vi "Add_APN.vi"(8 "error in (no error)":errorcluster, 11 "Add_APN":T1) -> (0 "error out":errorcluster, 3 "Output String":string)   [LabVIEW 2021]
uses:
  Controls/TCP_FGV.ctl
panel:
  # "SET,<add_apn>,<subscriber_N>,<no_of_apn>,<apn_name_i>,<qci_i>,<priority_level_i>,<no_of_dedicated_bearer_i_j>,<pcc_index_i_j>,<pcc_priority_index_i_j>,<mbr_dl_i_j>,<mbr_ul_i_j>,<gbr_dl_i_j>,<gbr_ul_i_j>"
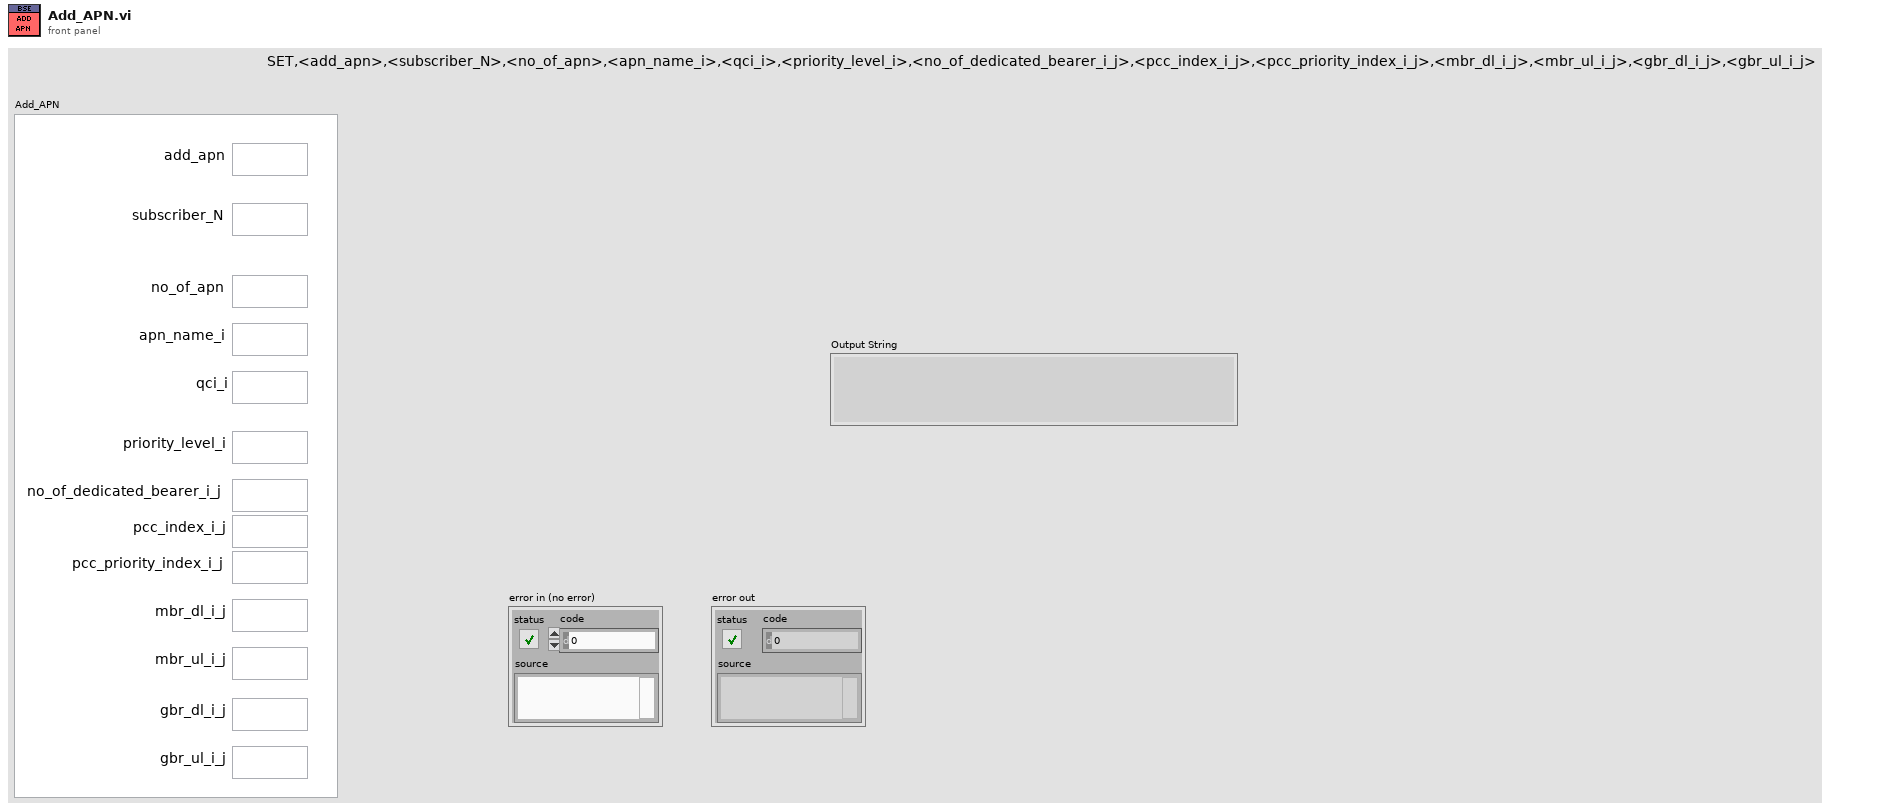
[diagram p1: front panel]
types:
  T1 = cluster{"add_apn":string, "subscriber_N":string, "no_of_apn":string, "apn_name_i":string, "qci_i":string, "priority_level_i":string, "no_of_dedicated_bearer_i_j":string, "pcc_index_i_j":string, "pcc_priority_index_i_j":string, "mbr_dl_i_j":string, "mbr_ul_i_j":string, "gbr_dl_i_j":string, "gbr_ul_i_j":string}
  T2 = typedef "TCP_FGV.ctl" = enum16{"Open", "Read", "Write", "Close"}
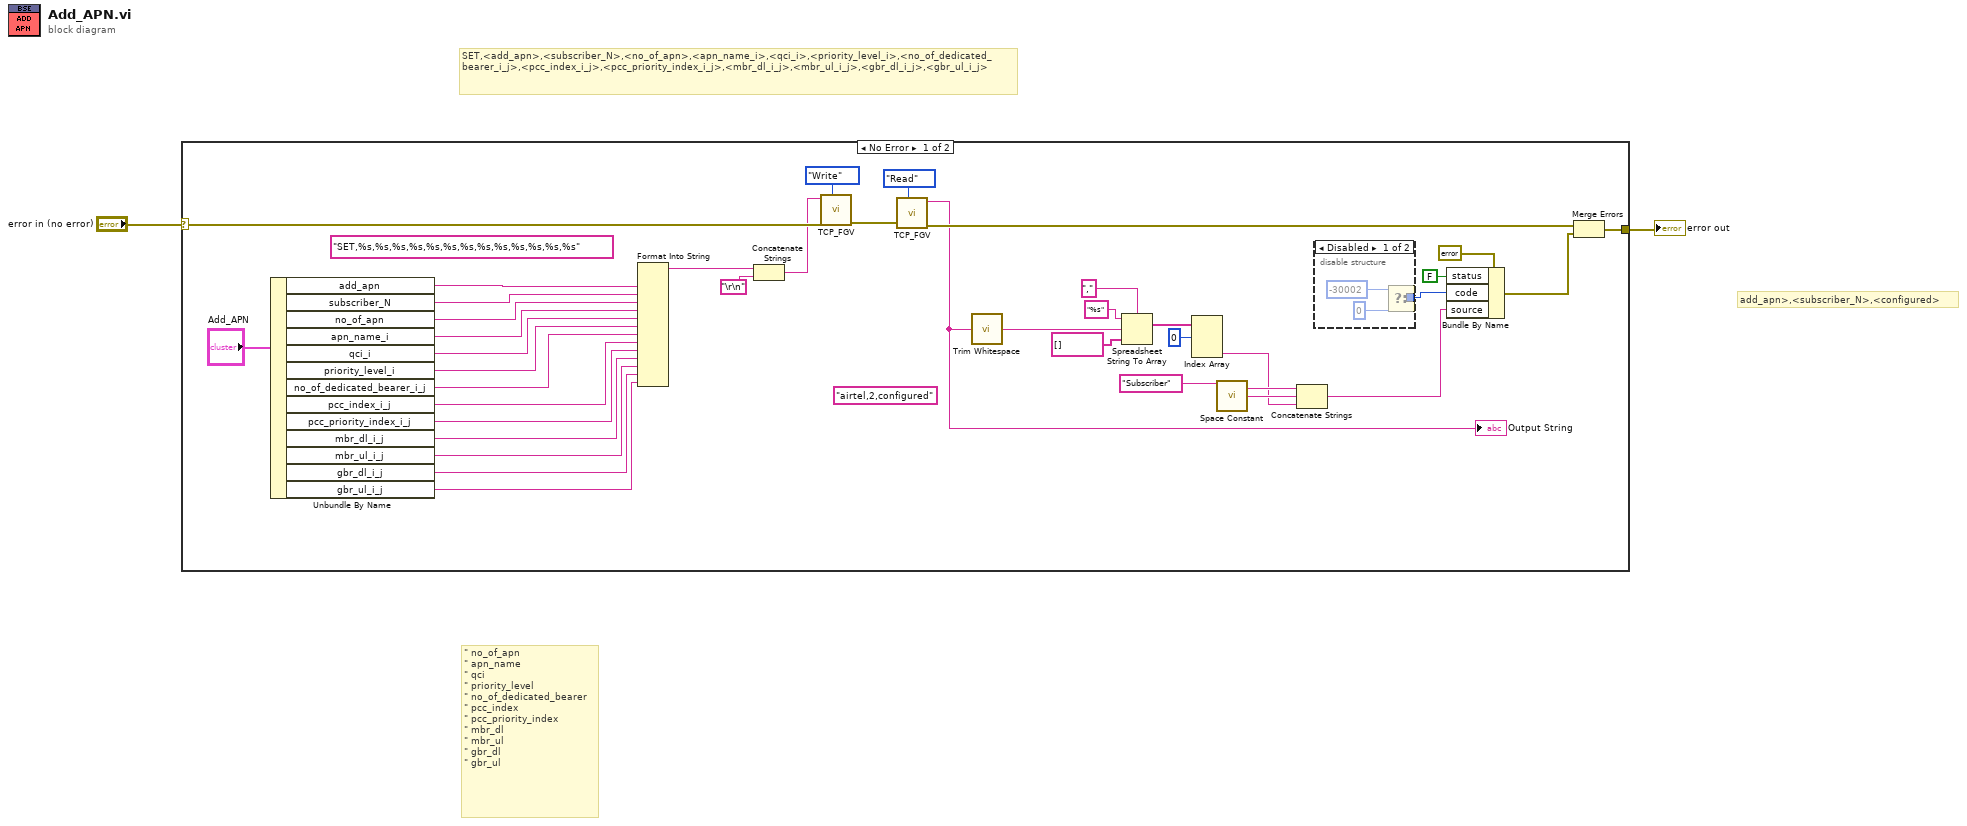
[diagram p0: block diagram]
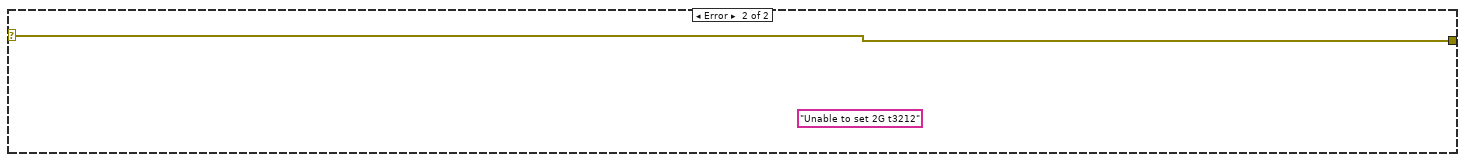
[diagram p3: hidden frame]
diagram:
  # "SET,<add_apn>,<subscriber_N>,<no_of_apn>,<apn_name_i>,<qci_i>,<priority_level_i>,<no_of_dedicated_bearer_i_j>,<pcc_index_i_j>,<pcc_priority_index_i_j>,<mbr_dl_i_j>,<mbr_ul_i_j>,<gbr_dl_i_j>,<gbr_ul_i_j>"
  # "\"\tno_of_apn \n\"\tapn_name\n\"\tqci\n\"\tpriority_level\n\"\tno_of_dedicated_bearer\n\"\tpcc_index\n\"\tpcc_priority_index\n\"\tmbr_dl\n\"\tmbr_ul\n\"\tgbr_dl\n\"\tgbr_ul"
  # "add_apn>,<subscriber_N>,<configured>"
  n1 = case shown="No Error" "error in (no error)" {
    selector: "error in (no error)" -> [w40 w44]
    tunnel: [w29 w44] -> w1
    frame No Error {
      (unwired) "airtel,2,configured" ("format string")
      (unwired) "SET,%s,%s,%s,%s,%s,%s,%s,%s,%s,%s,%s,%s,%s" ("format string")
      n2 = Unbundle By Name("Add_APN") -> ("add_apn"=w21:string, "subscriber_N"=w20:string, "no_of_apn"=w11:string, "apn_name_i"=w12:string, "qci_i"=w19:string, "priority_level_i"=w18:string, "no_of_dedicated_bearer_i_j"=w17:string, "pcc_index_i_j"=w9:string, "pcc_priority_index_i_j"=w8:string, "mbr_dl_i_j"=w7:string, "mbr_ul_i_j"=w6:string, "gbr_dl_i_j"=w5:string, "gbr_ul_i_j"=w4:string)
      n3 = Format Into String(w21, w20, w11, w12, w19, w18, w17, w9, w8, w7, w6, w5, w4) -> (resulting string=w25:string)  [unwired: 3 in, 1 out]
      n4 = Concatenate Strings(w25, "\r\n") -> (w24:string)
      n5 = call "TCP_FGV.vi"("Command"=w24, "error in (no error)"=w40, "Operation"=TCP_FGV."Write") -> ("error out"=w30:errorcluster)  [unwired: 6 in, 1 out]
      n6 = call "TCP_FGV.vi"("error in (no error)"=w30, "Operation"=TCP_FGV."Read") -> ("Data Out"=w10:string, "error out"=w32:errorcluster)  [unwired: 7 in]
      "Output String" <- w10
      n7 = call <vilib>:"Trim Whitespace.vi"("string"=w10) -> ("trimmed string"=w38:string)  [unwired: 1 in]
      n8 = Spreadsheet String To Array(delimiter (Tab)=",", format string="%s", spreadsheet string=w38, array type (2D Dbl)=string[] []) -> (array=w37:string[])
      n9 = Index Array(array=w37, index #1=0 ("index")) -> (element #3=w13:string)  [unwired: 2 in, 2 out]
      n10 = call <vilib>:"Space Constant.vi"() -> ("String"=w15:string)
      n11 = Concatenate Strings("Subscriber" ("format string"), w15, w13) -> (w28:string)
      n12 = disable-structure shown="Disabled" {
        disable-tunnel: [w43 _] -> w39
        frame Disabled {
          n13 = Select(t=-30002 ("code"), f=0 ("code")) -> (s? t:f=w43:i32)  [unwired: 1 in]
        }
        frame Enabled {
        }
      }
      n14 = Bundle By Name(cluster=errorcluster {"status"=FALSE, "code"=0, "source"=""} ("error constant"), "status"=FALSE, "code"=w39, "source"=w28) -> (w31:errorcluster)
      n15 = Merge Errors(w32, w31) -> (w29:errorcluster)
    }
    frame Error {
      (unwired) "Unable to set 2G t3212" ("source")
    }
  }
  "error out" <- w1
